vi "Read fit_Lower_Bound.vi"(8 "error in (no error)":errorcluster, 11 "Plots in":refnum<class "Plots.lvclass">) -> (0 "error out":errorcluster, 2 "fit_Lower_Bound":dbl[](array[numeric]), 3 "Plots out":refnum<class "Plots.lvclass">)   [LabVIEW 2018, in "Plots.lvclass"]
uses:
  Plots.lvclass
  Plots.lvclass/Plots.ctl
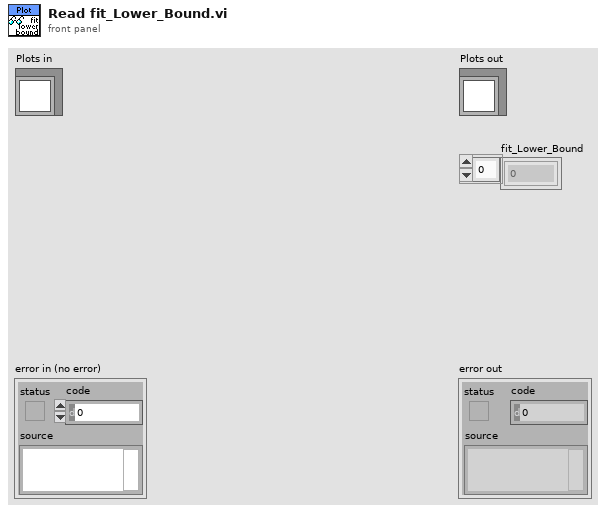
[diagram p1: front panel]
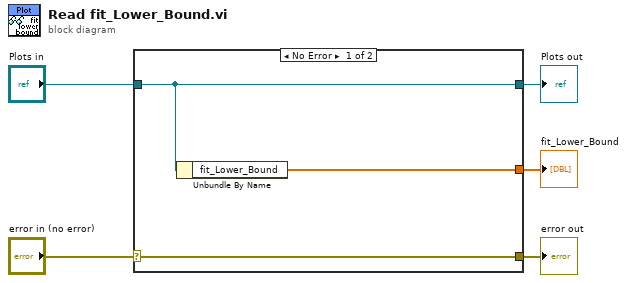
[diagram p0: block diagram]
diagram:
  n1 = case shown="No Error" "error in (no error)" {
    selector: "error in (no error)" -> [w8 w9]
    tunnel: [w8 w9] -> w4
    tunnel: [w7 w10] -> w2
    tunnel: "Plots in" -> [w7 w10]
    tunnel: [w6 _] -> w1
    frame No Error {
      n2 = Unbundle By Name(w7) -> ("fit_Lower_Bound"=w6:dbl[])
    }
    frame Error {
    }
  }
  "error out" <- w4
  "Plots out" <- w2
  "fit_Lower_Bound" <- w1
